vi "Read Spectrogram Time.vi"(8 "error in (no error)":errorcluster, 11 "VISA resource name":refnum<visa-resource-name>) -> (0 "error out":errorcluster, 1 "Time Stamp":dbl, 2 "Number Of Seconds":dbl, 3 "VISA resource name out":refnum<visa-resource-name>)   [LabVIEW 2016, in "Tektronix DPO MSO 2000 4000 Series.lvlib"]
doc: "Reads the time in the spectrogram.\n\n<B>Notes:</B>\nThis VI is available for MDO models only."
uses:
  Tektronix DPO MSO 2000 4000 Series.lvlib
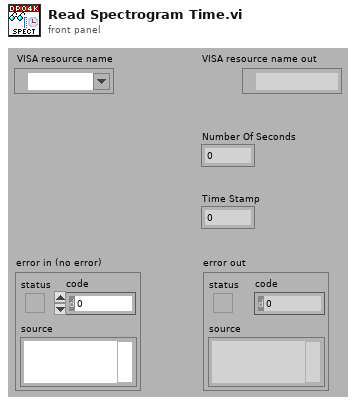
[diagram p1: front panel]
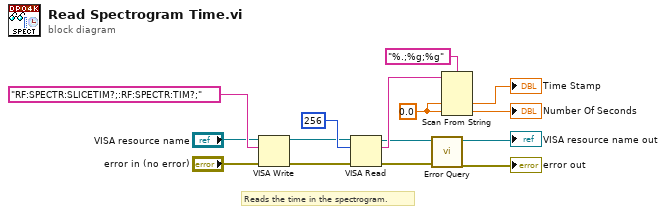
[diagram p0: block diagram]
diagram:
  w11 = 0.0 ("default value 1")
  # "Reads the time in the spectrogram."
  n1 = VISA Write(VISA resource name="VISA resource name", write buffer="RF:SPECTR:SLICETIM?;:RF:SPECTR:TIM?;", error in (no error)="error in (no error)") -> (VISA resource name out=w2:refnum<visa-resource-name>, error out=w1:errorcluster)  [unwired: 1 out]
  n2 = VISA Read(VISA resource name=w2, byte count=u32 256, error in (no error)=w1) -> (VISA resource name out=w4:refnum<visa-resource-name>, read buffer=w10:string, error out=w3:errorcluster)  [unwired: 1 out]
  n3 = call "Error Query.vi"("error in (no error)"=w3, "VISA resource name"=w4) -> ("error out"=→"error out":errorcluster, "VISA resource name out"=→"VISA resource name out":refnum<visa-resource-name>)  [unwired: 6 in, 2 out]
  n4 = Scan From String(format string="%.;%g;%g", input string=w10, default 1=w11, default 2=w11) -> (output 1=→"Time Stamp":dbl, output 2=→"Number Of Seconds":dbl)  [unwired: 2 in, 3 out]
